vi "Curve Editor.vi"(11 "OpenFile":bool) -> (8 "文件路径":path)   [LabVIEW 2020, in "Curve Editor.lvlib"]
uses:
  Curve Editor.lvlib
  <vilib>/Utility/miscctls.llb/LVPointTypeDef.ctl
  <vilib>/Utility/file.llb/Read From Spreadsheet File (string).vi
  Key Value/Key Value.lvlib
panel:
  in  "Exit":bool
  out "总时长[秒]":dbl format="%.2f"
  out "曲线预览":cluster{"X":dbl[], "Y":dbl[]}(graph)
  out "操作队列":refnum<queue>
  out "文件参数":T1
  out "选中的标识符":string
  out "复制的数据数组":string[](array[string])
  in  "粘贴组按钮":bool
  in  "复制组按钮":bool
  in  "编辑组按钮":bool
  in  "删除组按钮":bool
  in  "添加组按钮":bool
  in  "新建按钮":bool
  in  "另存为按钮":bool
  in  "保存按钮":bool
  in  "打开按钮":bool
  in  "循环树形":string(tree) caption="循环编辑"
  in  "动作列表框":i32(listbox) caption="曲线片段"
  out "颜色符号列表":cluster{"项名":string, "颜色":u32, "符号":i32}[](array[cluster])
  out "存盘提醒":bool
  out "读取文件":refnum<user-event>
  in  "文件_窗体标题":string="流程编辑"
  out "保存文件":refnum<user-event>
  out "文件已保存":bool
  out "双击行:缩进层次":i32
  in  "循环数组":string[](array[string])
  out "删除的行数":i32
  out "删除起始行索引":i32
  out "初始化":refnum<user-event>
  out "删除成功":bool
  out "删除行索引":i32
  out "添加成功":bool
  out "添加行索引":i32
  out "符号数组":picture[](array[picture])
  out "双击行":i32
  # "曲线编辑"
  # "组操作"
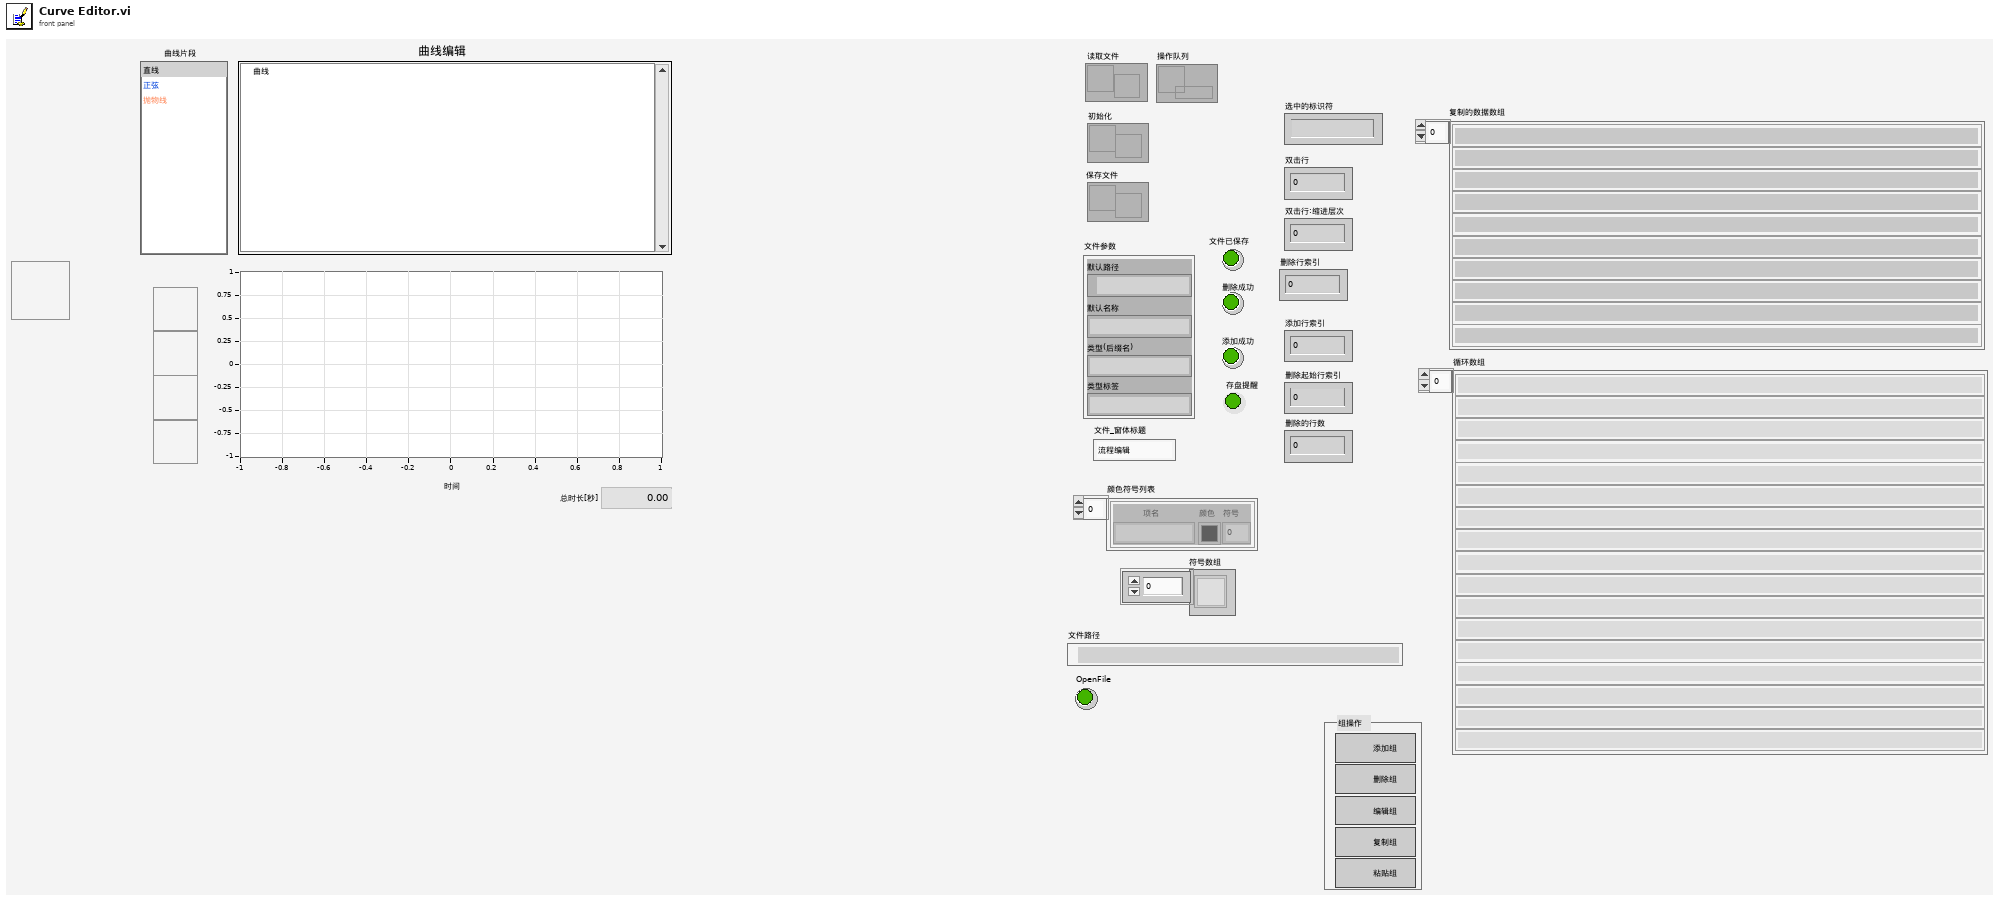
[diagram p1: front panel]
types:
  T1 = cluster{"默认路径":path, "默认名称":string, "类型(后缀名)":string, "类型标签":string}
  T2 = enum16{"Left Button", "Center Button", "Right Button", "Window Close"}
  T3 = typedef "LVPointTypeDef.ctl" = cluster{"Horizontal":i16, "Vertical":i16}
  T4 = cluster{"开始路径":path, "默认名称":string, "类型(后缀名)":string, "类型标签":string}
  T5 = enum16{"open", "replace", "create", "open or create", "replace or create", "replace or create with confirmation"}
  T6 = typedef "LVPoint32TypeDef.ctl" = cluster{"Horizontal":i32, "Vertical":i32}
  T7 = enum32{"invalid app kind", "Development System", "Run Time System", "Student Edition", "Embedded LabVIEW", "Evaluation", "Custom"}
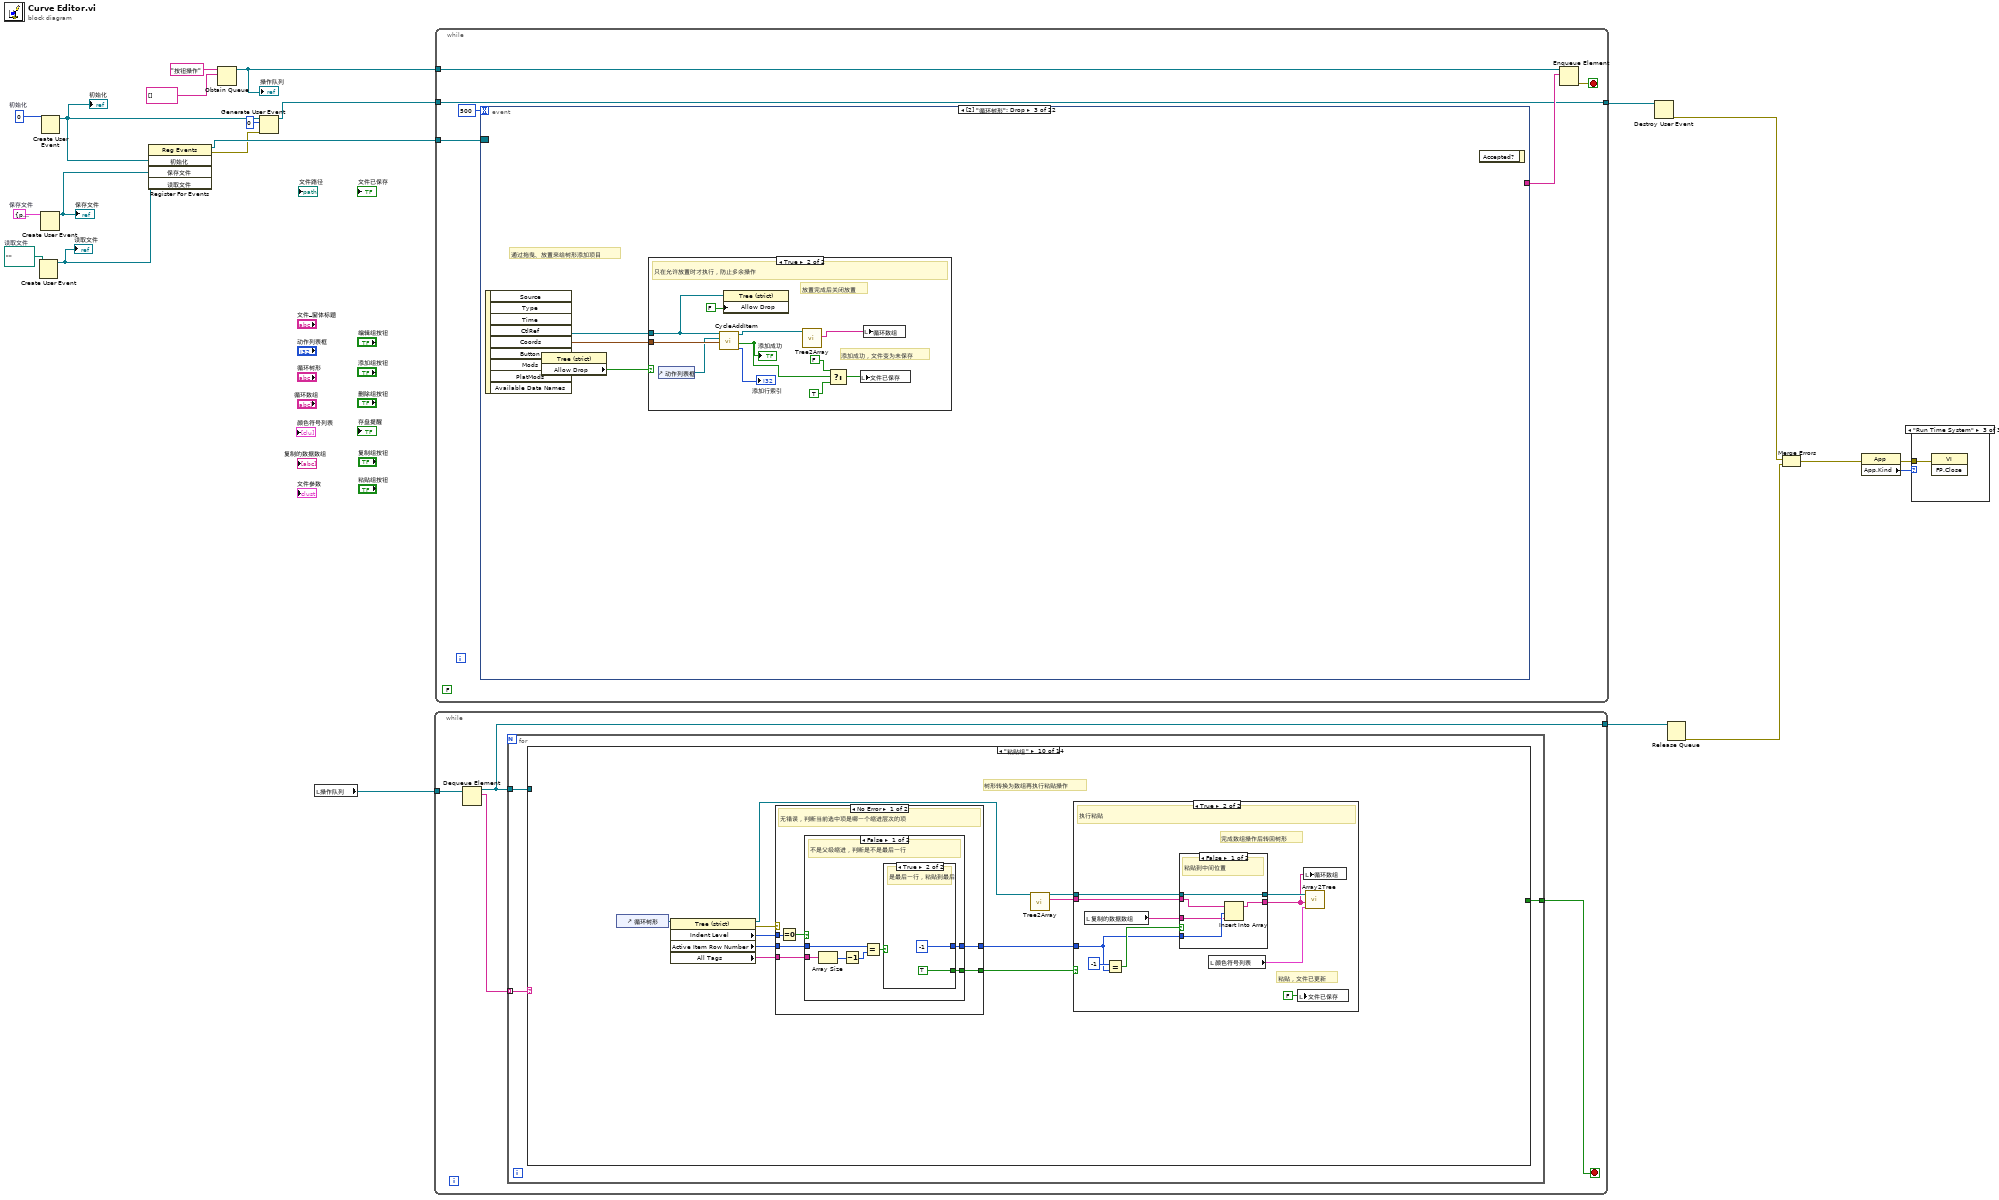
[diagram p0: block diagram]
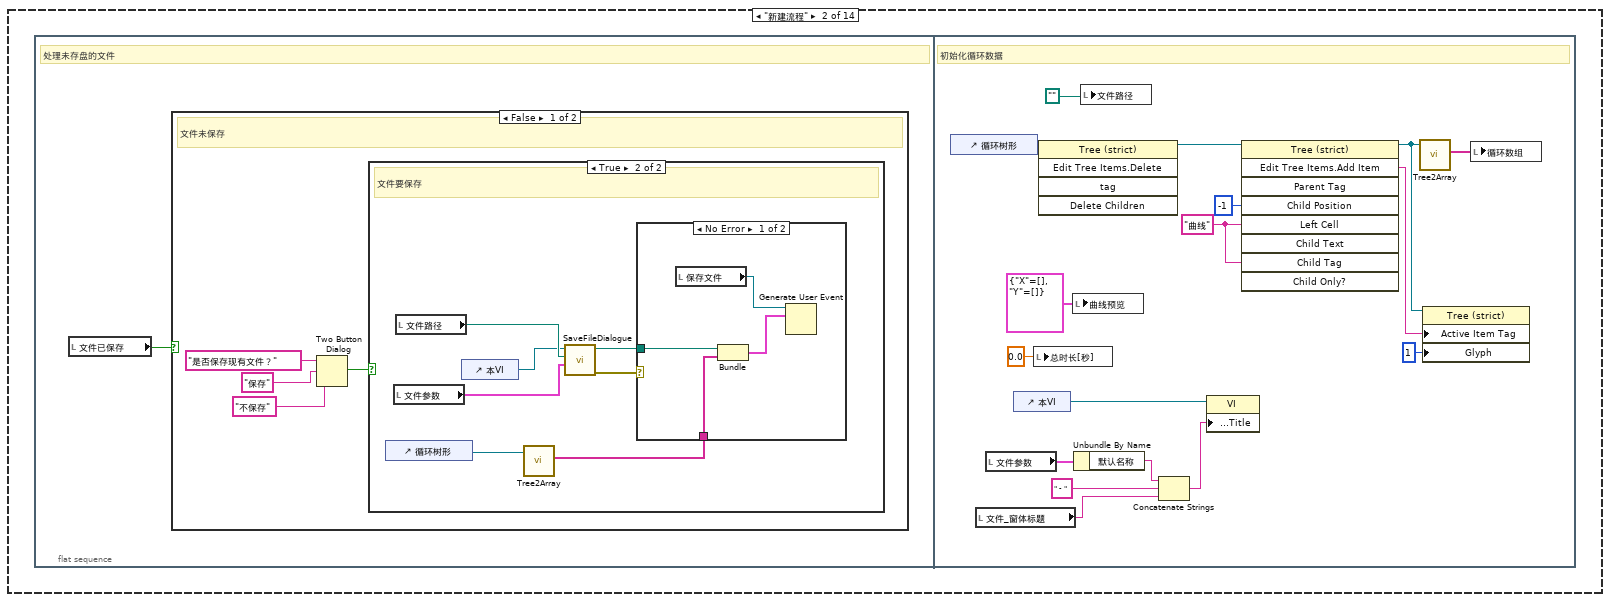
[diagram p5: hidden frame]
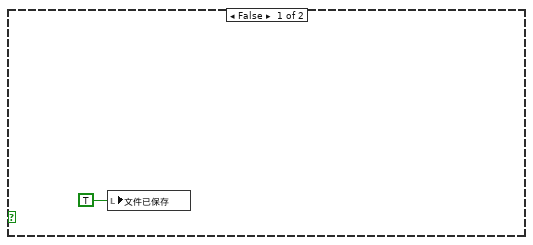
[diagram p6: hidden frame]
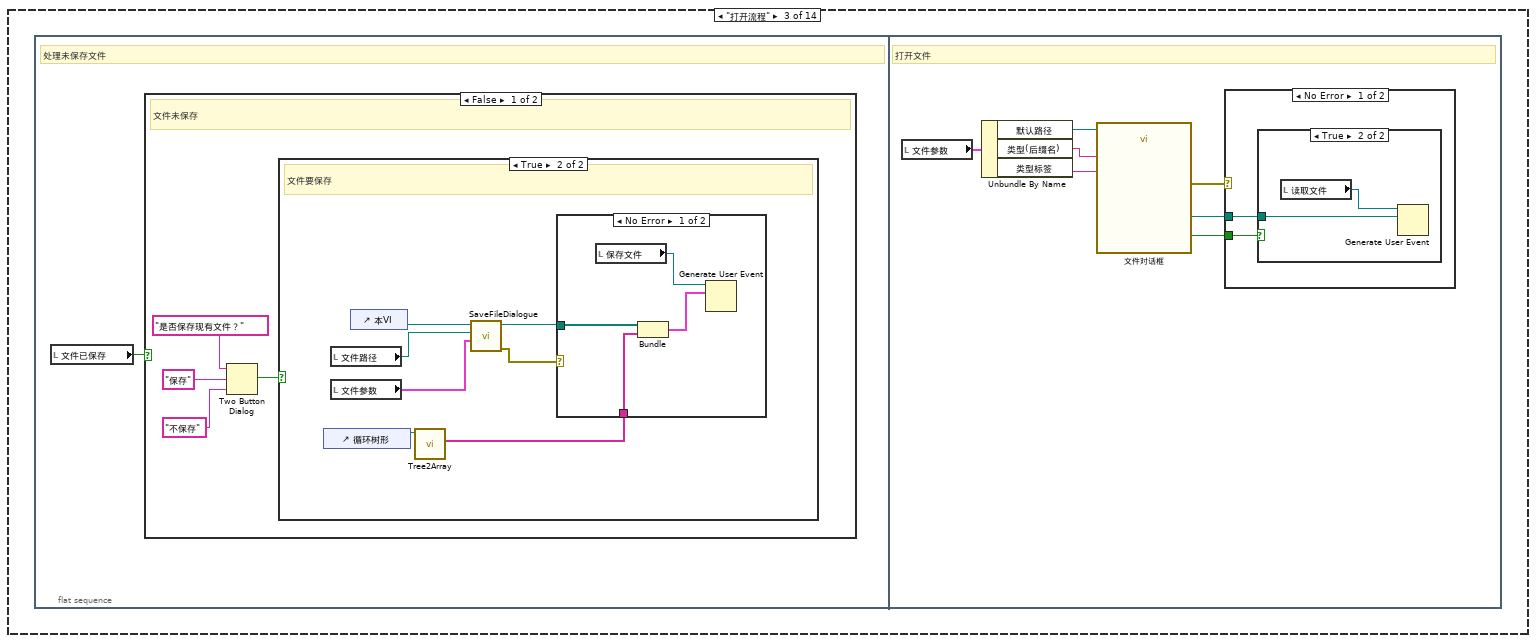
[diagram p9: hidden frame]
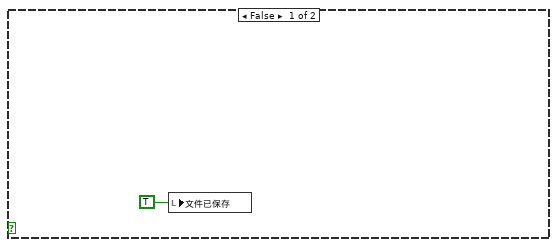
[diagram p10: hidden frame]
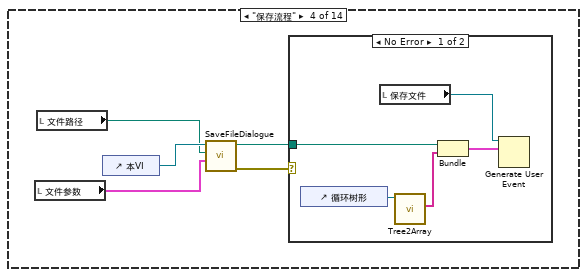
[diagram p15: hidden frame]
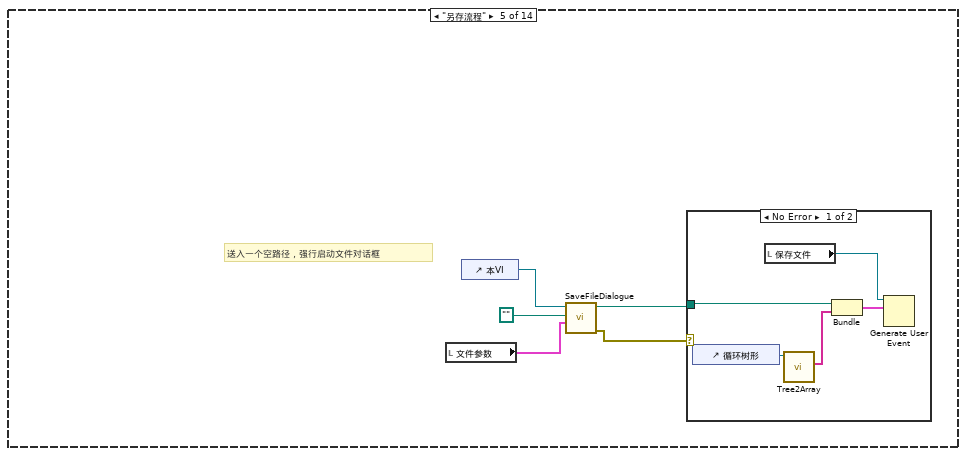
[diagram p17: hidden frame]
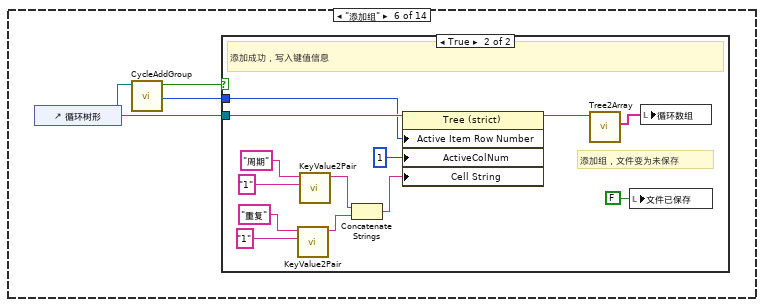
[diagram p19: hidden frame]
diagram:
  w14 = path ""  # 读取文件
  w15 = cluster{"路径":path, "数据":string[]} {"路径"=path "", "数据"=[]}  # 保存文件
  w21 = 0  # 初始化
  n1 = Create User Event(user event datatype=w14) -> (user event=w13:refnum<user-event>)  [unwired: 1 in, 1 out]
  "读取文件" <- w13
  n2 = Create User Event(user event datatype=w15) -> (user event=w16:refnum<user-event>)  [unwired: 1 in, 1 out]
  "保存文件" <- w16
  n3 = Create User Event(user event datatype=w21) -> (user event=w18:refnum<user-event>)  [unwired: 1 in, 1 out]
  "初始化" <- w18
  n4 = register-events(w18, w16, w13) -> (reference out=w20:refnum<event-registration>, error out=w17:errorcluster)  [unwired: 2 in]
  n5 = Obtain Queue(name (unnamed)="按钮操作" ("名称（未命名）"), element data type=string[] []) -> (queue out=w10:refnum<queue>)  [unwired: 3 in, 2 out]
  "操作队列" <- w10
  n6 = Generate User Event(user event=w18, event data cluster=0 ("事件数据"), error in=w17) -> (user event out=w7:refnum<user-event>)  [unwired: 1 in, 1 out]
  n7 = local read "操作队列"() -> (w9:refnum<queue>)
  n8 = while {
    tunnel: w9 -> [w25]
    tunnel: [w22] -> w8
    stop <- w23 stop-if-true
    n9 = Dequeue Element(queue=w25) -> (queue out=w22:refnum<queue>, element=w24:string[])  [unwired: 2 in, 2 out]
    n10 = for {
      tunnel: w22 -> [w28]
      tunnel: w24 -> [w27] mode=indexing
      tunnel: [w26] -> w23
      n11 = case shown="\"粘贴组\"" w27 {
        tunnel: w28 -> [_ _ _ _ _ _ _ _ _ _ _ _ _ _]
        tunnel: [_ _ _ _ _ _ _ _ _ _ _ _ _ w286] -> w26
        frame "假", Default {
        }
        frame "新建流程" {
          n12 = flat-sequence {
            frame #0 {
              # "处理未存盘的文件"
              n13 = local read "文件已保存"() -> (w29:bool)
              n14 = case shown="False" w29 {
                frame False {
                  # "文件未保存"
                  n15 = Two Button Dialog(message="是否保存现有文件？" ("消息"), 1:"不保存" ("F按钮名称（“取消”）"), 2:"保存" ("T按钮名称（“确定”）")) -> (T button?=w32:bool)
                  n16 = case shown="True" w32 {
                    frame False {
                      n17 = local write "文件已保存"(TRUE ("新建按钮")) -> ()
                    }
                    frame True {
                      # "文件要保存"
                      n18 = control-ref of="循环树形"() -> (w38:refnum<vi>)
                      n19 = local read "文件参数"() -> (w35:T1)
                      n20 = local read "文件路径"() -> (w41:path)
                      n21 = control-ref of="本VI"() -> (w36:refnum<vi>)
                      n22 = call "Tree2Array.vi"("TreeControl输入"=w38) -> ("循环数组"=w37:string[])  [unwired: 9 in, 1 out]
                      n23 = call "SaveFileDialogue.vi"("文件参数"=w35, "文件路径"=w41, "VI输入"=w36) -> ("错误输出"=w40:errorcluster, "输出路径"=w39:path)  [unwired: 6 in, 1 out]
                      n24 = case shown="No Error" w40 {
                        tunnel: w39 -> [w44 _]
                        tunnel: w37 -> [w42 _]
                        frame No Error {
                          n25 = local read "保存文件"() -> (w45:refnum<user-event>)
                          n26 = Bundle("输出路径"=w44, "循环数组"=w42) -> (w43:cluster{"输出路径":path, "循环数组":string[]})  [unwired: 1 in]
                          n27 = Generate User Event(user event=w45, event data cluster=w43) -> ()  [unwired: 2 in, 2 out]
                        }
                        frame Error {
                        }
                      }
                    }
                  }
                }
                frame True {
                  # "文件已保存"
                }
              }
            }
            frame #1 {
              w51 = "曲线" ("左单元格字符串")
              # "初始化循环数据"
              n28 = control-ref of="循环树形"() -> (w61:refnum<vi>)
              n29 = local read "文件_窗体标题"() -> (w59:string)
              n30 = local read "文件参数"() -> (w55:T1)
              n31 = control-ref of="本VI"() -> (w60:refnum<vi>)
              n32 = local write "总时长[秒]"(0.0 ("总时长[秒]")) -> ()
              n33 = invoke class="Tree (strict)" method="Edit Tree Items.Delete"(reference=w61) -> (reference out=w53:refnum<vi>)  [unwired: 4 in, 4 out]
              n34 = local write "曲线预览"(cluster{"X":dbl[], "Y":dbl[]} {"X"=[], "Y"=[]} ("曲线预览")) -> ()
              n35 = Unbundle By Name(w55) -> ("默认名称"=w54:string)
              n36 = local write "文件路径"(path "") -> ()
              n37 = Concatenate Strings(w54, " - " ("字符串"), w59) -> (w57:string)
              n38 = property class="VI"(reference=w60, "Front Panel.Title"=w57) -> ()  [unwired: 1 in, 2 out]
              n39 = invoke class="Tree (strict)" method="Edit Tree Items.Add Item"(reference=w53, "Child Position"=-1 ("子项位置"), "Left Cell"=w51, "Child Tag"=w51) -> (reference out=w50:refnum<vi>, "Edit Tree Items:Add Item"=w49:string)  [unwired: 5 in, 7 out]
              n40 = call "Tree2Array.vi"("TreeControl输入"=w50) -> ("循环数组"=w56:string[])  [unwired: 9 in, 1 out]
              n41 = property class="Tree (strict)"(reference=w50, "Active Item Tag"=w49, "Glyph"=1 ("活动项:符号索引")) -> ()  [unwired: 1 in, 2 out]
              n42 = local write "循环数组"(w56) -> ()
            }
          }
        }
        frame "打开流程" {
          n43 = flat-sequence {
            frame #0 {
              # "处理未保存文件"
              n44 = local read "文件已保存"() -> (w63:bool)
              n45 = case shown="False" w63 {
                frame False {
                  # "文件未保存"
                  n46 = Two Button Dialog(message="是否保存现有文件？" ("消息"), 1:"不保存" ("F按钮名称（“取消”）"), 2:"保存" ("T按钮名称（“确定”）")) -> (T button?=w66:bool)
                  n47 = case shown="True" w66 {
                    frame False {
                      n48 = local write "文件已保存"(TRUE ("新建按钮")) -> ()
                    }
                    frame True {
                      # "文件要保存"
                      n49 = control-ref of="循环树形"() -> (w75:refnum<vi>)
                      n50 = local read "文件路径"() -> (w72:path)
                      n51 = local read "文件参数"() -> (w71:T1)
                      n52 = control-ref of="本VI"() -> (w73:refnum<vi>)
                      n53 = call "Tree2Array.vi"("TreeControl输入"=w75) -> ("循环数组"=w74:string[])  [unwired: 9 in, 1 out]
                      n54 = call "SaveFileDialogue.vi"("文件参数"=w71, "文件路径"=w72, "VI输入"=w73) -> ("错误输出"=w70:errorcluster, "输出路径"=w69:path)  [unwired: 6 in, 1 out]
                      n55 = case shown="No Error" w70 {
                        tunnel: w69 -> [w78 _]
                        tunnel: w74 -> [w76 _]
                        frame No Error {
                          n56 = local read "保存文件"() -> (w79:refnum<user-event>)
                          n57 = Bundle("输出路径"=w78, "循环数组"=w76) -> (w77:cluster{"输出路径":path, "循环数组":string[]})  [unwired: 1 in]
                          n58 = Generate User Event(user event=w79, event data cluster=w77) -> ()  [unwired: 2 in, 2 out]
                        }
                        frame Error {
                        }
                      }
                    }
                  }
                }
                frame True {
                  # "文件已保存"
                }
              }
            }
            frame #1 {
              # "打开文件"
              n59 = local read "文件参数"() -> (w83:T1)
              n60 = Unbundle By Name(w83) -> ("默认路径"=w82:path, "类型(后缀名)"=w81:string, "类型标签"=w80:string)
              n61 = call "文件对话框"("start path"=w82, "pattern (all files)"=w81, "pattern label"=w80) -> ("selected path"=w84:path, "exists"=w86:bool, "error out"=w85:errorcluster)  [unwired: 9 in, 1 out]
              n62 = case shown="No Error" w85 {
                tunnel: w84 -> [w87 _]
                tunnel: w86 -> [w88 _]
                frame No Error {
                  n63 = case shown="True" w88 {
                    tunnel: w87 -> [_ w89]
                    frame False {
                    }
                    frame True {
                      n64 = local read "读取文件"() -> (w90:refnum<user-event>)
                      n65 = Generate User Event(user event=w90, event data cluster=w89) -> ()  [unwired: 2 in, 2 out]
                    }
                  }
                }
                frame Error {
                }
              }
            }
          }
        }
        frame "保存流程" {
          n66 = local read "文件参数"() -> (w93:T1)
          n67 = local read "文件路径"() -> (w91:path)
          n68 = control-ref of="本VI"() -> (w92:refnum<vi>)
          n69 = call "SaveFileDialogue.vi"("文件参数"=w93, "文件路径"=w91, "VI输入"=w92) -> ("错误输出"=w95:errorcluster, "输出路径"=w94:path)  [unwired: 6 in, 1 out]
          n70 = case shown="No Error" w95 {
            tunnel: w94 -> [w100 _]
            frame No Error {
              n71 = control-ref of="循环树形"() -> (w98:refnum<vi>)
              n72 = local read "保存文件"() -> (w99:refnum<user-event>)
              n73 = call "Tree2Array.vi"("TreeControl输入"=w98) -> ("循环数组"=w96:string[])  [unwired: 9 in, 1 out]
              n74 = Bundle("输出路径"=w100, "循环数组"=w96) -> (w97:cluster{"输出路径":path, "循环数组":string[]})  [unwired: 1 in]
              n75 = Generate User Event(user event=w99, event data cluster=w97) -> ()  [unwired: 2 in, 2 out]
            }
            frame Error {
            }
          }
        }
        frame "另存流程" {
          # "送入一个空路径，强行启动文件对话框"
          n76 = local read "文件参数"() -> (w102:T1)
          n77 = control-ref of="本VI"() -> (w101:refnum<vi>)
          n78 = call "SaveFileDialogue.vi"("文件参数"=w102, "文件路径"=path "", "VI输入"=w101) -> ("错误输出"=w104:errorcluster, "输出路径"=w103:path)  [unwired: 6 in, 1 out]
          n79 = case shown="No Error" w104 {
            tunnel: w103 -> [w110 _]
            frame No Error {
              n80 = control-ref of="循环树形"() -> (w108:refnum<vi>)
              n81 = local read "保存文件"() -> (w109:refnum<user-event>)
              n82 = call "Tree2Array.vi"("TreeControl输入"=w108) -> ("循环数组"=w106:string[])  [unwired: 9 in, 1 out]
              n83 = Bundle("输出路径"=w110, "循环数组"=w106) -> (w107:cluster{"输出路径":path, "循环数组":string[]})  [unwired: 1 in]
              n84 = Generate User Event(user event=w109, event data cluster=w107) -> ()  [unwired: 2 in, 2 out]
            }
            frame Error {
            }
          }
        }
        frame "添加组" {
          n85 = control-ref of="循环树形"() -> (w113:refnum<vi>)
          n86 = call "CycleAddGroup.vi"("TreeControl输入"=w113) -> ("添加的索引"=w111:i32, "添加成功"=w112:bool)  [unwired: 8 in, 1 out]
          n87 = case shown="True" w112 {
            tunnel: w111 -> [_ w122]
            tunnel: w113 -> [_ w126]
            frame False {
            }
            frame True {
              # "添加组，文件变为未保存"
              # "添加成功，写入键值信息"
              n88 = call "KeyValue2Pair.vi"("值"="1", "键"="重复") -> ("键值对"=w116:string)  [unwired: 9 in]
              n89 = call "KeyValue2Pair.vi"("值"="1", "键"="周期") -> ("键值对"=w115:string)  [unwired: 9 in]
              n90 = Concatenate Strings(w115, w116) -> (w114:string)
              n91 = property class="Tree (strict)"(reference=w126, "Active Item Row Number"=w122, "ActiveColNum"=1 ("活动单元格:活动列数"), "Cell String"=w114) -> (reference out=w121:refnum<vi>)  [unwired: 1 in, 1 out]
              n92 = call "Tree2Array.vi"("TreeControl输入"=w121) -> ("循环数组"=w119:string[])  [unwired: 9 in, 1 out]
              n93 = local write "文件已保存"(FALSE ("文件已保存")) -> ()
              n94 = local write "循环数组"(w119) -> ()
            }
          }
        }
        frame "删除组" {
          # "有行被删除，文件变为未保存"
          n95 = control-ref of="循环树形"() -> (w127:refnum<vi>)
          n96 = call "CycleRemoveGroup.vi"("TreeControl输入"=w127) -> ("删除的行数"=w130:i32, "删除起始行索引"=→"删除起始行索引":i32, "TreeControl输出"=w129:refnum<vi>)  [unwired: 8 in]
          "删除的行数" <- w130
          n97 = Greater Than 0?(x=w130) -> (x > 0?=w134:bool)
          n98 = call "Tree2Array.vi"("TreeControl输入"=w129) -> ("循环数组"=w135:string[])  [unwired: 9 in, 1 out]
          n99 = Select(t=FALSE, s=w134, f=TRUE) -> (s? t:f=w133:bool)
          n100 = local write "循环数组"(w135) -> ()
          n101 = local write "文件已保存"(w133) -> ()
        }
        frame "编辑组" {
          # "获取行索引和标识"
          n102 = control-ref of="循环树形"() -> (w140:refnum<vi>)
          n103 = property class="Tree (strict)" props=["Active Item Row Number", "Active Item Tag", "Indent Level", "All Tags"](reference=w140) -> (reference out=w137:refnum<vi>, error out=w136:errorcluster, "Active Item Row Number"=w139:i32, "Indent Level"=w138:i32)  [unwired: 1 in, 2 out]
          n104 = case shown="No Error" w136 {
            tunnel: w138 -> [w144 _]
            tunnel: w137 -> [w142 _]
            tunnel: w139 -> [w141 _]
            frame No Error {
              n105 = Equal To 0?(x=w144) -> (x = 0?=w143:bool)
              n106 = case shown="True" w143 {
                tunnel: w142 -> [_ w151]
                tunnel: w141 -> [_ w150]
                frame False {
                  n107 = One Button Dialog(message="请选择组！" ("消息")) -> ()  [unwired: 1 in, 1 out]
                }
                frame True {
                  # "编辑窗打开，文件变为未保存"
                  # "是组级索引时调用编辑窗"
                  n108 = vi-ref "EditGroup.vi"() -> (w149:refnum<vi>)
                  n109 = call "CallEditVI.vi"("VI引用句柄"=w149, "索引"=w150, "TreeControl输入"=w151) -> ("TreeControl输出"=w148:refnum<vi>)  [unwired: 7 in, 1 out]
                  n110 = call "Tree2Array.vi"("TreeControl输入"=w148) -> ("循环数组"=w146:string[])  [unwired: 9 in, 1 out]
                  n111 = local write "文件已保存"(FALSE) -> ()
                  n112 = local write "循环数组"(w146) -> ()
                }
              }
            }
            frame Error {
              n113 = One Button Dialog(message="请选择组！" ("消息")) -> ()  [unwired: 1 in, 1 out]
            }
          }
        }
        frame "复制组" {
          # "获取当前项行索引及缩进级别"
          n114 = control-ref of="循环树形"() -> (w153:refnum<vi>)
          n115 = property class="Tree (strict)"(reference=w153) -> (reference out=w157:refnum<vi>, error out=w155:errorcluster, "Indent Level"=w154:i32, "Active Item Row Number"=w156:i32)  [unwired: 1 in]
          n116 = case shown="No Error" w155 {
            tunnel: w154 -> [w161 _]
            tunnel: w156 -> [w159 _]
            tunnel: w157 -> [w158 _]
            frame No Error {
              n117 = Equal To 0?(x=w161) -> (x = 0?=w160:bool)
              n118 = case shown="True" w160 {
                tunnel: w159 -> [_ w167]
                tunnel: w158 -> [_ w170]
                frame False {
                  n119 = One Button Dialog(message="请选择组！" ("消息")) -> ()  [unwired: 1 in, 1 out]
                }
                frame True {
                  # "将索引指向下一项"
                  # "获取组信息"
                  n120 = call "TreeRow2String.vi"("类型"=enum16{"动作", "组"}."组", "索引"=w167, "TreeControl输入"=w170) -> ("键值串"=w166:string, "TreeControl输出"=w168:refnum<vi>)  [unwired: 7 in]
                  n121 = Increment(x=w167) -> (x+1=w163:i32)
                  n122 = Build Array(w166) -> (w165:string[])
                  n123 = while {
                    tunnel: w168 -> [w181]
                    shift-right: [w171] -> w164
                    shift-left: w165 -> [w172]
                    tunnel: w163 -> [w180]
                    i -> [w179]
                    stop <- w175 stop-if-true
                    # "遇到下一个父项或超出最后行时停止"
                    # "从父项后的一项开始遍历后面的各项"
                    n124 = Add(x=w180, y=w179) -> (x+y=w174:i32)
                    n125 = property class="Tree (strict)"(reference=w181, "Active Item Row Number"=w174) -> (reference out=w173:refnum<vi>, error out=w176:errorcluster, "Indent Level"=w177:i32)  [unwired: 1 in]
                    n126 = Equal To 0?(x=w177) -> (x = 0?=w178:bool)
                    n127 = Or(x=w176, y=w178) -> (x .or. y?=w175:bool)
                    n128 = case shown="False" w175 {
                      tunnel: w174 -> [w187 _]
                      tunnel: w173 -> [w186 _]
                      tunnel: w172 -> [w184 w188]
                      tunnel: [w182 w188] -> w171
                      frame False {
                        # "未遇到下一个父项或超出最后\n行时添加临时数组"
                        n129 = call "TreeRow2String.vi"("类型"=enum16{"动作", "组"}."动作", "索引"=w187, "TreeControl输入"=w186) -> ("键值串"=w183:string)  [unwired: 7 in, 1 out]
                        n130 = Build Array (concatenate)(w184, w183) -> (w182:string[])
                      }
                      frame True {
                      }
                    }
                  }
                  n131 = local write "复制的数据数组"(w164) -> ()
                }
              }
            }
            frame Error {
              n132 = One Button Dialog(message="请选择组！" ("消息")) -> ()  [unwired: 1 in, 1 out]
            }
          }
        }
        frame "粘贴组" {
          # "树形转换为数组再执行粘贴操作"
          n133 = control-ref of="循环树形"() -> (w190:refnum<vi>)
          n134 = property class="Tree (strict)"(reference=w190) -> (reference out=w197:refnum<vi>, error out=w192:errorcluster, "Indent Level"=w191:i32, "Active Item Row Number"=w193:i32, "All Tags"=w194:string[])  [unwired: 1 in]
          n135 = case shown="No Error" w192 {
            tunnel: w191 -> [w224 _]
            tunnel: w193 -> [w221 _]
            tunnel: w194 -> [w219 _]
            tunnel: [w220 -1] -> w195
            tunnel: [w222 TRUE] -> w196
            frame No Error {
              # "无错误，判断当前选中项是哪一个缩进层次的项"
              n136 = Equal To 0?(x=w224) -> (x = 0?=w223:bool)
              n137 = case shown="False" w223 {
                tunnel: [w226 TRUE] -> w222
                tunnel: [w225 w237] -> w220
                tunnel: w221 -> [w228 w237]
                tunnel: w219 -> [w231 _]
                frame False {
                  # "不是父级缩进，判断是不是最后一行"
                  n138 = Array Size(array=w231) -> (size(s)=w230:i32)
                  n139 = Decrement(x=w230) -> (x-1=w229:i32)
                  n140 = Equal?(x=w228, y=w229) -> (x = y?=w227:bool)
                  n141 = case shown="True" w227 {
                    tunnel: [FALSE TRUE] -> w226
                    tunnel: [-1 -1] -> w225
                    frame False {
                      # "不是最后行，提示\n不粘贴"
                      n142 = One Button Dialog(message="请选择组位置！" ("消息")) -> ()  [unwired: 1 in, 1 out]
                    }
                    frame True {
                      # "是最后一行，粘贴到最后"
                    }
                  }
                }
                frame True {
                  # "是父级缩进，在当前行插入"
                }
              }
            }
            frame Error {
              # "如果有错，直接往最后一行添加"
            }
          }
          n143 = call "Tree2Array.vi"("TreeControl输入"=w197) -> ("循环数组"=w199:string[], "TreeControl输出"=w198:refnum<vi>)  [unwired: 9 in]
          n144 = case shown="True" w196 {
            tunnel: w195 -> [_ w204]
            tunnel: w198 -> [_ w207]
            tunnel: w199 -> [_ w206]
            frame False {
              # "不执行粘贴"
            }
            frame True {
              # "粘贴，文件已更新"
              # "完成数组操作后转回树形"
              # "执行粘贴"
              n145 = local read "复制的数据数组"() -> (w205:string[])
              n146 = Equal?(x=-1, y=w204) -> (x = y?=w208:bool)
              n147 = case shown="False" w208 {
                tunnel: w207 -> [w210 w215]
                tunnel: w206 -> [w214 w218]
                tunnel: w205 -> [w212 w217]
                tunnel: [w211 w216] -> w201
                tunnel: w204 -> [w213 _]
                tunnel: [w210 w215] -> w203
                frame False {
                  # "粘贴到中间位置"
                  n148 = Insert Into Array(array=w214, index=w213, new element=w212) -> (w211:string[])
                }
                frame True {
                  # "粘贴到最后一行"
                  n149 = Build Array (concatenate)(w218, w217) -> (w216:string[])
                }
              }
              n150 = local read "颜色符号列表"() -> (w202:cluster{"项名":string, "颜色":u32, "符号":i32}[])
              n151 = local write "文件已保存"(FALSE ("文件已保存")) -> ()
              n152 = local write "循环数组"(w201) -> ()
              n153 = call "Array2Tree.vi"("颜色符号列表"=w202, "循环数组"=w201, "循环树形引用输入"=w203) -> ()  [unwired: 7 in, 2 out]
            }
          }
        }
        frame "编辑项" {
          # "通过标识获取行索引和首列文本"
          n154 = control-ref of="循环树形"() -> (w241:refnum<vi>)
          n155 = property class="Tree (strict)"(reference=w241, "ActiveColNum"=0 ("活动单元格:活动列数")) -> (reference out=w245:refnum<vi>, error out=w244:errorcluster, "Active Item Row Number"=w246:i32, "Indent Level"=w247:i32, "Cell String"=w243:string)  [unwired: 1 in]
          "双击行" <- w246
          "双击行:缩进层次" <- w247
          n156 = case shown="No Error" w244 {
            selector: w244 -> [_ w268]
            tunnel: w243 -> [w254 _]
            tunnel: w245 -> [w253 _]
            tunnel: w246 -> [w252 _]
            tunnel: w247 -> [w251 _]
            frame No Error {
              n157 = Not Equal To 0?(x=w251) -> (x != 0?=w250:bool)
              n158 = case shown="True" w250 {
                tunnel: w254 -> [_ w263]
                tunnel: w253 -> [_ w262]
                tunnel: w252 -> [_ w259]
                tunnel: [string[] [] ("元素") string[] ["绘制曲线"] ("元素")] -> w248
                frame False {
                }
                frame True {
                  # "编辑窗打开，文件变为未保存"
                  # "打开编辑窗口"
                  # "动作选择"
                  # "当为子项时打开编辑窗口"
                  n159 = case shown="\"假\", Default" w263 {
                    tunnel: [w264 w265 w266 w267] -> w260
                    frame "假", Default {
                      (unwired) refnum<vi> refnum
                      n160 = vi-ref "EditLine.vi"() -> (w264:refnum<vi>)
                    }
                    frame "直线" {
                      n161 = vi-ref "EditLine.vi"() -> (w265:refnum<vi>)
                    }
                    frame "正弦" {
                      n162 = vi-ref "EditSine.vi"() -> (w266:refnum<vi>)
                    }
                    frame "抛物线" {
                      n163 = vi-ref "EditParabola.vi"() -> (w267:refnum<vi>)
                    }
                  }
                  n164 = call "CallEditVI.vi"("VI引用句柄"=w260, "索引"=w259, "TreeControl输入"=w262) -> ("TreeControl输出"=w261:refnum<vi>)  [unwired: 7 in, 1 out]
                  n165 = local write "文件已保存"(FALSE ("文件已保存")) -> ()
                  n166 = call "Tree2Array.vi"("TreeControl输入"=w261) -> ("循环数组"=w257:string[])  [unwired: 9 in, 1 out]
                  n167 = local write "循环数组"(w257) -> ()
                }
              }
              n168 = local read "操作队列"() -> (w249:refnum<queue>)
              n169 = Enqueue Element(queue=w249, element=w248) -> ()  [unwired: 2 in, 3 out]
            }
            frame Error {
              n170 = call <vilib>:"Clear Errors.vi"("error in (no error)"=w268) -> ()  [unwired: 5 in, 2 out]
            }
          }
        }
        frame "绘制曲线" {
          n171 = control-ref of="循环树形"() -> (w275:refnum<vi>)
          n172 = call "Tree2Array.vi"("TreeControl输入"=w275) -> ("循环数组"=w274:string[])  [unwired: 9 in, 1 out]
          n173 = call "DrawCurve.vi"("曲线定义数组"=w274) -> ("曲线输出"=w273:cluster{"X":dbl[], "Y":dbl[]})  [unwired: 10 in]
          "曲线预览" <- w273
          n174 = Unbundle(w273) -> ("X"=w271:dbl[])  [unwired: 1 out]
          n175 = Delete From Array(array=w271, length=1 ("长度")) -> (deleted portion=w270:dbl[])  [unwired: 1 in, 1 out]
          n176 = Index Array(array=w270) -> (element=→"总时长[秒]":dbl)  [unwired: 1 in]
        }
        frame "删除项" {
          n177 = flat-sequence {
            frame #0 {
              # "删除成功，文件变为未保存"
              # "通过拖曳删除动作"
              n178 = control-ref of="循环树形"() -> (w276:refnum<vi>)
              n179 = call "CycleRemoveItem.vi"("TreeControl输入"=w276) -> ("删除行索引"=→"删除行索引":i32, "删除成功"=w279:bool, "TreeControl输出"=w278:refnum<vi>)  [unwired: 8 in]
              "删除成功" <- w279
              n180 = call "Tree2Array.vi"("TreeControl输入"=w278) -> ("循环数组"=w283:string[])  [unwired: 9 in, 1 out]
              n181 = local write "循环数组"(w283) -> ()
              n182 = Select(t=FALSE, s=w279, f=TRUE) -> (s? t:f=w282:bool)
              n183 = local write "文件已保存"(w282) -> ()
            }
            frame #1 {
              n184 = local read "操作队列"() -> (w284:refnum<queue>)
              n185 = Enqueue Element(queue=w284, element=string[] ["绘制曲线"] ("元素")) -> ()  [unwired: 2 in, 3 out]
            }
          }
        }
        frame "退出" {
          n186 = local read "文件已保存"() -> (w288:bool)
          n187 = case shown="False" w288 {
            tunnel: [w289 FALSE] -> w287
            frame False {
              n188 = call <vilib>:"Three Button Dialog.vi"("Window Title (\"\")"="关闭窗口" ("Window Title (\"\")"), "Center Button Text (\"No\")"="不保存" ("Center Button Text (\"No\")"), "Left Button Text (\"Yes\")"="保存" ("Left Button Text (\"Yes\")"), "message"="是否保存当前文件？") -> ("Which Button?"=w290:T2)  [unwired: 7 in]
              n189 = case shown="\"Left Button\", Default" w290 {
                tunnel: [w295 FALSE TRUE TRUE] -> w289
                frame "Left Button", Default {
                  n190 = local write "存盘提醒"(FALSE ("存盘提醒")) -> ()
                  n191 = control-ref of="循环树形"() -> (w303:refnum<vi>)
                  n192 = control-ref of="本VI"() -> (w300:refnum<vi>)
                  n193 = local read "文件路径"() -> (w299:path)
                  n194 = local read "文件参数"() -> (w298:T1)
                  n195 = call "SaveFileDialogue.vi"("文件参数"=w298, "文件路径"=w299, "VI输入"=w300) -> ("错误输出"=w297:errorcluster, "取消"=w295:bool, "输出路径"=w296:path)  [unwired: 6 in]
                  n196 = call "Tree2Array.vi"("TreeControl输入"=w303) -> ("循环数组"=w301:string[])  [unwired: 9 in, 1 out]
                  n197 = case shown="No Error" w297 {
                    tunnel: w296 -> [w306 _]
                    tunnel: w301 -> [w304 _]
                    frame No Error {
                      n198 = local read "保存文件"() -> (w307:refnum<user-event>)
                      n199 = Bundle("输出路径"=w306, "循环数组"=w304) -> (w305:cluster{"输出路径":path, "循环数组":string[]})  [unwired: 1 in]
                      n200 = Generate User Event(user event=w307, event data cluster=w305) -> ()  [unwired: 2 in, 2 out]
                    }
                    frame Error {
                    }
                  }
                }
                frame "Center Button" {
                }
                frame "Right Button" {
                }
                frame "Window Close" {
                }
              }
            }
            frame True {
            }
          }
          n201 = Not(x=w287) -> (.not. x?=w286:bool)
        }
      }
    }
  }
  n202 = while {
    tunnel: w20 -> [w317]
    tunnel: w10 -> [w316]
    tunnel: [w314] -> w6
    tunnel: w7 -> [w314]
    stop <- w313 stop-if-true
    (unwired) FALSE
    n203 = event shown="[2] \"循环树形\": Drop" {
      selector: w317 -> [_ _ _ _ _ _ _ _ _ _ _ _ _ _ _ _ _ _ _ _ _ _]
      dyn-events: _ -> [_ _ _ _ _ _ _ _ _ _ _ _ _ _ _ _ _ _ _ _ _ _]
      timeout: 500 -> [_ _ _ _ _ _ _ _ _ _ _ _ _ _ _ _ _ _ _ _ _ _]
      tunnel: [_ _ _ string[] ["删除项"] ("元素") string[] ["新建流程"] ("元素") w337 _ _ string[] ["退出"] ("元素") string[] ["复制组"] ("元素") string[] ["粘贴组"] ("元素") string[] ["保存流程"] ("元素") string[] ["另存流程"] ("元素") _ _ string[] ["退出"] ("元素") w460 string[] ["打开流程"] ("元素") string[] ["添加组"] ("元素") string[] ["删除组"] ("元素") string[] ["编辑组"] ("元素") _] -> w315
      event Timeout {
        n204 = event-data() -> ()  [unwired: 1 in, 3 out]
      }
      event "动作列表框": Drag Starting {
        # "拖曳开始时，允许树形接受放置"
        n205 = event-data() -> ()  [unwired: 1 in, 10 out]
        n206 = control-ref of="循环树形"() -> (w319:refnum<vi>)
        n207 = property class="Tree (strict)"(reference=w319, "Allow Drop"=TRUE ("拖曳/放置:允许放置")) -> ()  [unwired: 1 in, 2 out]
      }
      event "循环树形": Drop {
        # "通过拖曳、放置来给树形添加项目"
        n208 = event-data() -> ("CtlRef"=w320:refnum<vi>, "Coords"=w322:T6)  [unwired: 1 in, 7 out]
        n209 = property class="Tree (strict)"(reference=w320) -> ("Allow Drop"=w321:bool)  [unwired: 1 in, 2 out]
        n210 = case shown="True" w321 {
          tunnel: w322 -> [_ w333]
          tunnel: w320 -> [_ w330]
          frame False {
          }
          frame True {
            # "添加成功，文件变为未保存"
            # "放置完成后关闭放置"
            # "只在允许放置时才执行，防止多余操作"
            n211 = control-ref of="动作列表框"() -> (w332:refnum<vi>)
            n212 = call "CycleAddItem.vi"("Coords"=w333, "动作列表框"=w332, "TreeControl输入"=w330) -> ("添加行索引"=→"添加行索引":i32, "添加成功"=w324:bool, "TreeControl输出"=w329:refnum<vi>)  [unwired: 6 in]
            "添加成功" <- w324
            n213 = property class="Tree (strict)"(reference=w330, "Allow Drop"=FALSE ("拖曳/放置:允许放置")) -> ()  [unwired: 1 in, 2 out]
            n214 = call "Tree2Array.vi"("TreeControl输入"=w329) -> ("循环数组"=w323:string[])  [unwired: 9 in, 1 out]
            n215 = Select(t=FALSE, s=w324, f=TRUE) -> (s? t:f=w325:bool)
            n216 = local write "文件已保存"(w325) -> ()
            n217 = local write "循环数组"(w323) -> ()
          }
        }
        n218 = event-data() -> ()  [unwired: 2 in, 1 out]
      }
      event "循环树形": Drag Ended {
        n219 = event-data() -> ()  [unwired: 1 in, 5 out]
      }
      event "新建按钮": Value Change {
        n220 = event-data() -> ()  [unwired: 1 in, 6 out]
      }
      event "循环树形": Double Click {
        # "通过双击编辑项目"
        n221 = event-data() -> ("Coords"=w336:T6)  [unwired: 1 in, 9 out]
        n222 = flat-sequence {
          tunnel: w336 -> [w341]
          tunnel: [string[] ["编辑项"] ("元素")] -> w337
          frame #0 {
            # "定位到选中的标识"
            # "通过坐标获取标识"
            n223 = control-ref of="循环树形"() -> (w342:refnum<vi>)
            n224 = invoke class="Tree (strict)" method="Point To Row Column"(reference=w342, "Point"=w341) -> (reference out=w340:refnum<vi>, "Tag"=w339:string)  [unwired: 6 in, 6 out]
            n225 = property class="Tree (strict)"(reference=w340, "Active Item Tag"=w339) -> (error out=w338:errorcluster)  [unwired: 1 in, 1 out]
            n226 = call <vilib>:"Clear Errors.vi"("error in (no error)"=w338) -> ()  [unwired: 5 in, 2 out]
          }
          frame #1 {
          }
        }
      }
      event "循环树形": Drag Starting {
        w344 = FALSE ("添加成功")
        # "这里可删除"
        n227 = event-data() -> ()  [unwired: 1 in, 10 out]
        n228 = local write "删除成功"(w344) -> ()
        n229 = local write "添加成功"(w344) -> ()
      }
      event User Event {
        n230 = event-data() -> ()  [unwired: 1 in, 5 out]
        n231 = flat-sequence {
          frame #0 {
            w346 = u32 13816530
            w360 = TRUE ("文件已保存")
            w361 = "曲线编辑" ("前面板窗口:标题")
            w358 = string[] [] ("循环数组")
            w352 = FALSE ("添加组")
            # "树形清空"
            # "文件定义"
            n232 = control-ref of="循环树形"() -> (w367:refnum<vi>)
            n233 = control-ref of="窗格"() -> (w349:refnum<vi>)
            n234 = control-ref of="循环树形"() -> (w347:refnum<vi>)
            n235 = control-ref of="动作列表框"() -> (w365:refnum<vi>)
            n236 = control-ref of="本VI"() -> (w362:refnum<vi>)
            n237 = call <vilib>:"Application Directory.vi"() -> ("Application Directory"=w345:path)
            n238 = property class="Pane"(reference=w349, "Origin"=T3 {"Horizontal"=0, "Vertical"=0} ("原点")) -> ()  [unwired: 1 in, 2 out]
            n239 = call "InitializeCurveList.vi"("循环树形"=w347, "ListBox输入"=w365) -> ("符号数组"=→"符号数组":picture[], "颜色符号列表"=w359:cluster{"项名":string, "颜色":u32, "符号":i32}[], "Tree引用输出"=w363:refnum<vi>)  [unwired: 6 in, 1 out]
            n240 = local write "循环数组"(w358) -> ()
            n241 = local write "复制的数据数组"(w358) -> ()
            n242 = property class="Tree (strict)"(reference=w367, "Allow Drop"=FALSE ("拖曳/放置:允许放置")) -> ()  [unwired: 1 in, 2 out]
            n243 = property class="Tree (strict)"(reference=w347, "SelColor"=w346) -> ()  [unwired: 1 in, 2 out]
            n244 = property class="VI"(reference=w362, "Front Panel.Title"=w361) -> ()  [unwired: 1 in, 2 out]
            n245 = local write "文件_窗体标题"(w361) -> ()
            n246 = local write "颜色符号列表"(w359) -> ()
            n247 = Bundle By Name(cluster=T4 {"开始路径"=path "", "默认名称"="", "类型(后缀名)"="", "类型标签"=""} ("文件参数"), "开始路径"=w345, "默认名称"="新曲线" ("文件_默认文件名"), "类型(后缀名)"="*.cuv" ("文件_后缀名"), "类型标签"="曲线配置文件" ("文件_类型标签")) -> (w353:T4)
            n248 = invoke class="Tree (strict)" method="Edit Tree Items.Delete"(reference=w363) -> ()  [unwired: 4 in, 5 out]
            n249 = local write "曲线预览"(cluster{"X":dbl[], "Y":dbl[]} {"X"=[], "Y"=[]} ("曲线预览")) -> ()
            n250 = local write "文件参数"(w353) -> ()
            n251 = local write "添加组按钮"(w352) -> ()
            n252 = local write "删除组按钮"(w352) -> ()
            n253 = local write "编辑组按钮"(w352) -> ()
            n254 = local write "复制组按钮"(w352) -> ()
            n255 = local write "粘贴组按钮"(w352) -> ()
            n256 = local write "总时长[秒]"(0.0 ("总时长[秒]")) -> ()
            n257 = local write "文件已保存"(w360) -> ()
            n258 = local write "存盘提醒"(w360) -> ()
            n259 = property on="动作列表框" class="LstBox (strict)"("SelColor"=w346) -> ()  [unwired: 2 in, 2 out]
          }
          frame #1 {
            n260 = case shown="True" "OpenFile" {
              frame False {
              }
              frame True {
                n261 = local read "文件路径"() -> (w370:path)
                n262 = call <vilib>:"Is Path and Not Empty.vi"("path"=w370) -> ("Is Path and Not Empty?"=w369:bool)  [unwired: 4 in]
                n263 = case shown="True" w369 {
                  tunnel: w370 -> [_ w371]
                  frame False {
                  }
                  frame True {
                    n264 = local read "读取文件"() -> (w372:refnum<user-event>)
                    n265 = Generate User Event(user event=w372, event data cluster=w371) -> ()  [unwired: 2 in, 2 out]
                  }
                }
              }
            }
          }
        }
      }
      event "Exit": Value Change {
        n266 = event-data() -> ()  [unwired: 1 in, 6 out]
      }
      event "复制组按钮": Value Change {
        n267 = event-data() -> ()  [unwired: 1 in, 6 out]
        n268 = local write "复制组按钮"(FALSE ("复制组按钮")) -> ()
      }
      event "粘贴组按钮": Value Change {
        n269 = event-data() -> ()  [unwired: 1 in, 6 out]
        n270 = local write "粘贴组按钮"(FALSE ("粘贴组按钮")) -> ()
      }
      event "保存按钮": Value Change {
        n271 = event-data() -> ()  [unwired: 1 in, 6 out]
      }
      event "另存为按钮": Value Change {
        n272 = event-data() -> ()  [unwired: 1 in, 6 out]
      }
      event User Event {
        n273 = event-data() -> ("路径"=w380:path, "数据"=w387:string[])  [unwired: 1 in, 4 out]
        n274 = for {
          tunnel: w387 -> [w405] mode=indexing
          shift-right: [w402] -> w385
          shift-left: "" -> [w403]
          i -> [w410]
          # "将字符串数组转换为换行符分隔的字符串"
          n275 = Equal To 0?(x=w410) -> (x = 0?=w409:bool)
          n276 = Select(t="", s=w409, f="\n") -> (s? t:f=w406:string)
          n277 = Concatenate Strings(w406, w405) -> (w404:string)
          n278 = Concatenate Strings(w403, w404) -> (w402:string)
        }
        n279 = Open/Create/Replace File(file path (use dialog)=w380, operation (0:open)=T5."replace or create" ("操作(0:open)"), access (0:read/write)=enum16{"read/write", "read-only", "write-only"}."write-only" ("权限(0:read/write)")) -> (refnum out=w389:refnum<file>, error out=w388:errorcluster)  [unwired: 3 in, 1 out]
        n280 = Write to Text File(file (use dialog)=w389, text=w385, error in=w388) -> (refnum out=w384:refnum<file>, error out=w383:errorcluster)  [unwired: 1 in, 1 out]
        n281 = Close File(refnum=w384, error in=w383) -> (path=w381:path, error out=w382:errorcluster)
        n282 = case shown="No Error" w382 {
          tunnel: w381 -> [w395 _]
          frame No Error {
            n283 = local read "文件_窗体标题"() -> (w394:string)
            n284 = local write "文件路径"(w395) -> ()
            n285 = call <vilib>:"Get File Extension.vi"("file"=w395) -> ("filename without extension"=w397:string)  [unwired: 6 in, 4 out]
            n286 = local read "存盘提醒"() -> (w392:bool)
            n287 = local write "文件已保存"(TRUE ("文件已保存")) -> ()
            n288 = case shown="True" w392 {
              frame False {
              }
              frame True {
                n289 = One Button Dialog(message="文件保存成功！" ("消息")) -> ()  [unwired: 1 in, 1 out]
              }
            }
            n290 = control-ref of="本VI"() -> (w396:refnum<vi>)
            n291 = Concatenate Strings(w397, " - " ("字符串"), w394) -> (w399:string)
            n292 = property class="VI"(reference=w396, "Front Panel.Title"=w399) -> ()  [unwired: 1 in, 2 out]
          }
          frame Error {
            n293 = One Button Dialog(message="文件保存失败！" ("消息")) -> ()  [unwired: 1 in, 1 out]
          }
        }
      }
      event User Event {
        n294 = event-data() -> ("读取文件"=w414:path)  [unwired: 1 in, 4 out]
        n295 = call-poly <vilib>:"Read From Spreadsheet File.vi"("file path (dialog if empty)"=w414) -> ("all rows"=w420:string[][])  [unwired: 6 in, 4 out]
        n296 = local read "颜色符号列表"() -> (w416:cluster{"项名":string, "颜色":u32, "符号":i32}[])
        n297 = control-ref of="循环树形"() -> (w418:refnum<vi>)
        n298 = Index Array(array=w420, index (col)=0 ("禁用的索引 (列)")) -> (element=w417:string[])  [unwired: 1 in]
        n299 = call "Array2Tree.vi"("颜色符号列表"=w416, "循环数组"=w417, "循环树形引用输入"=w418) -> ("错误输出"=w415:errorcluster, "循环树形引用输出"=w413:refnum<vi>)  [unwired: 7 in]
        n300 = case shown="No Error" w415 {
          tunnel: w414 -> [w424 _]
          tunnel: w413 -> [w423 _]
          tunnel: [string[] ["绘制曲线"] ("元素") string[] [] ("元素")] -> w411
          frame No Error {
            n301 = call "Tree2Array.vi"("TreeControl输入"=w423) -> ("循环数组"=w422:string[])  [unwired: 9 in, 1 out]
            n302 = local read "文件_窗体标题"() -> (w426:string)
            n303 = local write "文件已保存"(TRUE ("文件已保存")) -> ()
            n304 = local write "文件路径"(w424) -> ()
            n305 = call <vilib>:"Get File Extension.vi"("file"=w424) -> ("filename without extension"=w428:string)  [unwired: 6 in, 4 out]
            n306 = local write "循环数组"(w422) -> ()
            n307 = control-ref of="本VI"() -> (w427:refnum<vi>)
            n308 = Concatenate Strings(w428, " - " ("字符串"), w426) -> (w430:string)
            n309 = property class="VI"(reference=w427, "Front Panel.Title"=w430) -> ()  [unwired: 1 in, 2 out]
          }
          frame Error {
          }
        }
        n310 = local read "操作队列"() -> (w412:refnum<queue>)
        n311 = Enqueue Element(queue=w412, element=w411) -> ()  [unwired: 2 in, 3 out]
      }
      event Panel Close? {
        n312 = event-data() -> ()  [unwired: 1 in, 4 out]
        n313 = disable-structure shown="禁用" {
          disable-tunnel: [w434 _] -> _
          frame Disabled {
            n314 = local read "文件已保存"() -> (w435:bool)
            n315 = case shown="False" w435 {
              tunnel: [w436 TRUE] -> w434
              frame False {
                n316 = call <vilib>:"Three Button Dialog.vi"("Window Title (\"\")"="关闭窗口" ("Window Title (\"\")"), "Center Button Text (\"No\")"="不保存" ("Center Button Text (\"No\")"), "Left Button Text (\"Yes\")"="保存" ("Left Button Text (\"Yes\")"), "message"="是否保存当前文件？") -> ("Which Button?"=w437:T2)  [unwired: 7 in]
                n317 = case shown="\"Left Button\", Default" w437 {
                  tunnel: [w442 FALSE FALSE TRUE] -> w436
                  frame "Left Button", Default {
                    n318 = local write "存盘提醒"(FALSE ("存盘提醒")) -> ()
                    n319 = control-ref of="循环树形"() -> (w451:refnum<vi>)
                    n320 = control-ref of="本VI"() -> (w448:refnum<vi>)
                    n321 = local read "文件路径"() -> (w447:path)
                    n322 = local read "文件参数"() -> (w446:T1)
                    n323 = call "SaveFileDialogue.vi"("文件参数"=w446, "文件路径"=w447, "VI输入"=w448) -> ("错误输出"=w445:errorcluster, "取消"=w443:bool, "输出路径"=w444:path)  [unwired: 6 in]
                    n324 = call "Tree2Array.vi"("TreeControl输入"=w451) -> ("循环数组"=w449:string[])  [unwired: 9 in, 1 out]
                    n325 = case shown="No Error" w445 {
                      tunnel: w444 -> [w454 _]
                      tunnel: w449 -> [w452 _]
                      frame No Error {
                        n326 = local read "保存文件"() -> (w455:refnum<user-event>)
                        n327 = Bundle("输出路径"=w454, "循环数组"=w452) -> (w453:cluster{"输出路径":path, "循环数组":string[]})  [unwired: 1 in]
                        n328 = Generate User Event(user event=w455, event data cluster=w453) -> ()  [unwired: 2 in, 2 out]
                      }
                      frame Error {
                      }
                    }
                    n329 = Not(x=w443) -> (.not. x?=w442:bool)
                  }
                  frame "Center Button" {
                  }
                  frame "Right Button" {
                  }
                  frame "Window Close" {
                  }
                }
              }
              frame True {
              }
            }
          }
          frame Enabled {
          }
        }
        n330 = event-data("Discard?"=TRUE ("放弃？")) -> ()  [unwired: 1 in, 1 out]
      }
      event Menu Selection (User) {
        n331 = event-data() -> ("ItemTag"=w461:string)  [unwired: 1 in, 6 out]
        n332 = case shown="\"退出\"" w461 {
          tunnel: [_ string[] ["退出"] ("元素") string[] ["新建流程"] ("元素") string[] ["编辑项"] ("元素") string[] ["删除项"] ("元素") string[] ["打开流程"] ("元素") string[] ["保存流程"] ("元素") string[] ["另存流程"] ("元素") string[] ["添加组"] ("元素") string[] ["删除组"] ("元素") string[] ["编辑组"] ("元素") string[] ["复制组"] ("元素") string[] ["粘贴组"] ("元素")] -> w460
          frame "假", Default {
          }
          frame "退出" {
          }
          frame "新建流程" {
          }
          frame "编辑项" {
          }
          frame "删除项" {
          }
          frame "打开流程" {
          }
          frame "保存流程" {
          }
          frame "另存流程" {
          }
          frame "添加组" {
          }
          frame "删除组" {
          }
          frame "编辑组" {
          }
          frame "复制组" {
          }
          frame "粘贴组" {
          }
        }
      }
      event "打开按钮": Value Change {
        n333 = event-data() -> ()  [unwired: 1 in, 6 out]
      }
      event "添加组按钮": Value Change {
        n334 = event-data() -> ()  [unwired: 1 in, 6 out]
        n335 = local write "添加组按钮"(FALSE ("添加组")) -> ()
      }
      event "删除组按钮": Value Change {
        n336 = event-data() -> ()  [unwired: 1 in, 6 out]
        n337 = local write "删除组按钮"(FALSE ("删除组")) -> ()
      }
      event "编辑组按钮": Value Change {
        n338 = event-data() -> ()  [unwired: 1 in, 6 out]
        n339 = local write "编辑组按钮"(FALSE ("重命名组")) -> ()
      }
      event "循环树形": Mouse Down {
        # "定位到前面获取的标识"
        # "通过坐标获取相应的标识"
        # "通过单击获取要编辑的项的标识，并定位到这个标识。是所有树形列表项操作的基础，十分重要"
        n340 = event-data() -> ("CtlRef"=w481:refnum<vi>, "Coords"=w482:T6)  [unwired: 1 in, 6 out]
        n341 = invoke class="Tree (strict)" method="Point To Row Column"(reference=w481, "Point"=w482) -> (reference out=w486:refnum<vi>, error out=w484:errorcluster, "Tag"=w485:string)  [unwired: 6 in, 5 out]
        "选中的标识符" <- w485
        n342 = property class="Tree (strict)"(reference=w486, error in=w484, "Active Item Tag"=w485) -> (error out=w483:errorcluster)  [unwired: 1 out]
        n343 = call <vilib>:"Clear Errors.vi"("error in (no error)"=w483) -> ()  [unwired: 5 in, 2 out]
      }
    }
    n344 = Enqueue Element(queue=w316, element=w315) -> (error out=w313:errorcluster)  [unwired: 2 in, 2 out]
  }
  n345 = Destroy User Event(user event=w6) -> (error out=w3:errorcluster)  [unwired: 1 in]
  n346 = Release Queue(queue=w8) -> (error out=w2:errorcluster)  [unwired: 2 in, 2 out]
  n347 = Merge Errors(w3, w2) -> (w1:errorcluster)
  n348 = property class="App"(error in=w1) -> (error out=w4:errorcluster, "App.Kind"=w5:T7)  [unwired: 1 in, 1 out]
  n349 = case shown="\"Run Time System\"" w5 {
    tunnel: w4 -> [_ _ w487]
    frame "invalid app kind", Default {
    }
    frame "Development System" {
    }
    frame "Run Time System" {
      n350 = invoke class="VI" method="FP.Close"(error in=w487) -> ()  [unwired: 2 in, 3 out]
    }
  }
